vi "Rotation Vectors.vi"(9 "Gyro Angle":dbl, 10 "upper limit":dbl, 11 "upper limit 2":dbl) -> (2 "X'":dbl, 3 "Y'":dbl)   [LabVIEW 2016]
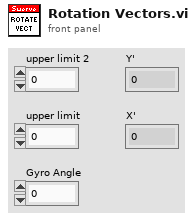
[diagram p1: front panel]
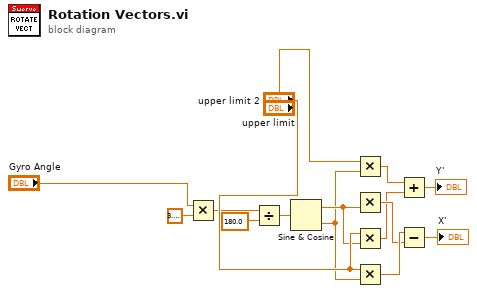
[diagram p0: block diagram]
diagram:
  n1 = Multiply(x="Gyro Angle", y=3.141592653589793) -> (x*y=w10:dbl)
  n2 = Divide(x=w10, y=180.0) -> (x/y=w9:dbl)
  n3 = Sine & Cosine(0:w9) -> (1:w5:dbl, 2:w4:dbl)
  n4 = Multiply(x="upper limit", y=w4) -> (x*y=w3:dbl)
  n5 = Multiply(y=w5) -> (x*y=w7:dbl)  [unwired: 1 in]
  n6 = Multiply(x="upper limit 2", y=w5) -> (x*y=w2:dbl)
  n7 = Multiply(x="upper limit 2", y=w4) -> (x*y=w8:dbl)
  n8 = Add(x=w3, y=w2) -> (x+y=→"Y'":dbl)
  n9 = Subtract(x=w8, y=w7) -> (x-y=→"X'":dbl)
